vi "FP_Origin.vi"(8 "error in":errorcluster, 10 "Origin":cluster{"Horizontal":i16, "Vertical":i16}, 11 "VI.Path":path) -> (0 "error out":errorcluster, 3 "VI Reference":refnum<vi>)   [LabVIEW 2015]
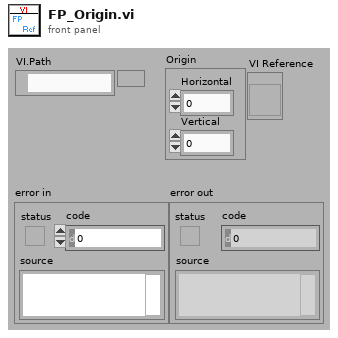
[diagram p1: front panel]
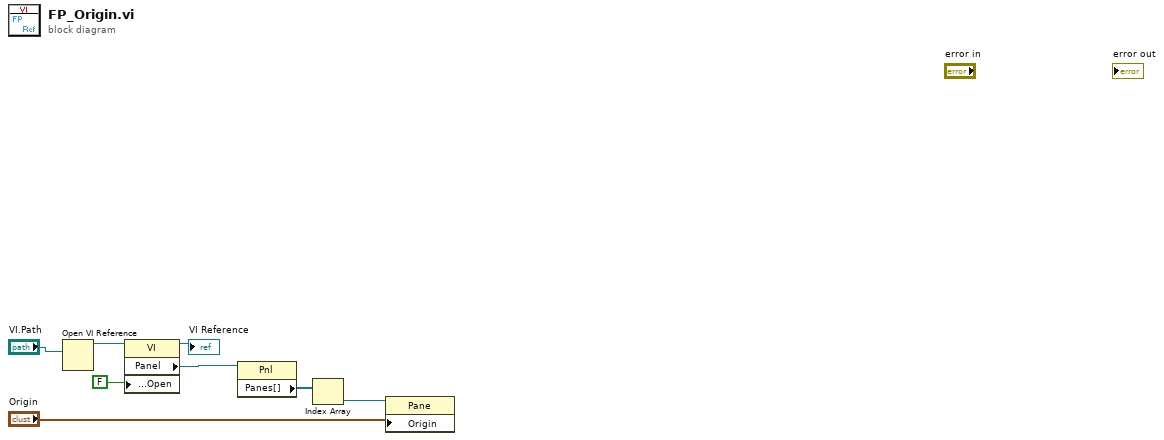
[diagram p0: block diagram]
diagram:
  n1 = Open VI Reference(vi path="VI.Path") -> (vi reference=w3:refnum<vi>)  [unwired: 5 in, 1 out]
  n2 = property class="VI"(reference=w3, "Front Panel.Open"=FALSE ("Front Panel Window:Open")) -> (reference out=→"VI Reference":refnum<vi>, "Panel"=w5:refnum<vi>)  [unwired: 1 in, 1 out]
  n3 = property class="Pnl"(reference=w5) -> ("Panes[]"=w6:refnum<vi>[])  [unwired: 1 in, 2 out]
  n4 = Index Array(array=w6) -> (element=w7:refnum<vi>)  [unwired: 1 in]
  n5 = property class="Pane"(reference=w7, "Origin"="Origin") -> ()  [unwired: 1 in, 2 out]
